vi "IsSearchGoalNode.vi"(8 "error in (no error)":errorcluster, 10 "PossibleGoalNode in":refnum<data-value>, 11 "Graph in":refnum<class "Graph.lvclass">) -> (0 "error out":errorcluster, 1 "IsGoal":bool, 2 "PossibleGoalNode out":refnum<data-value>, 3 "Graph out":refnum<class "Graph.lvclass">)   [LabVIEW 2010, in "Graph.lvclass"]
doc: "Abstract method. Override this VI to implement a search of a tree. This VI is responsible for determining when we have found the node we are searching for."
uses:
  Graph.lvclass
  GraphNode/GraphNode.lvclass
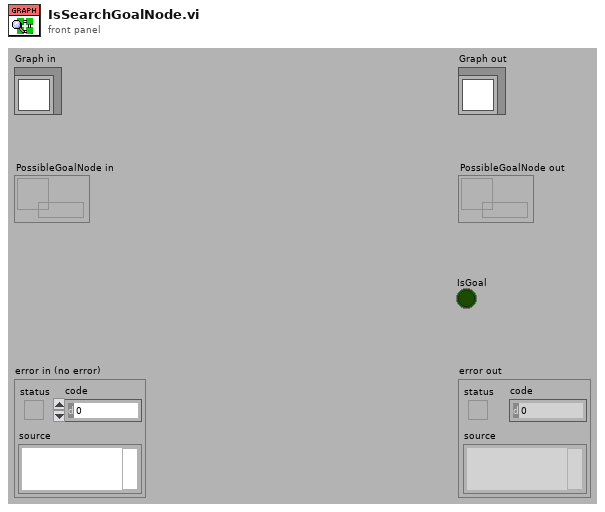
[diagram p1: front panel]
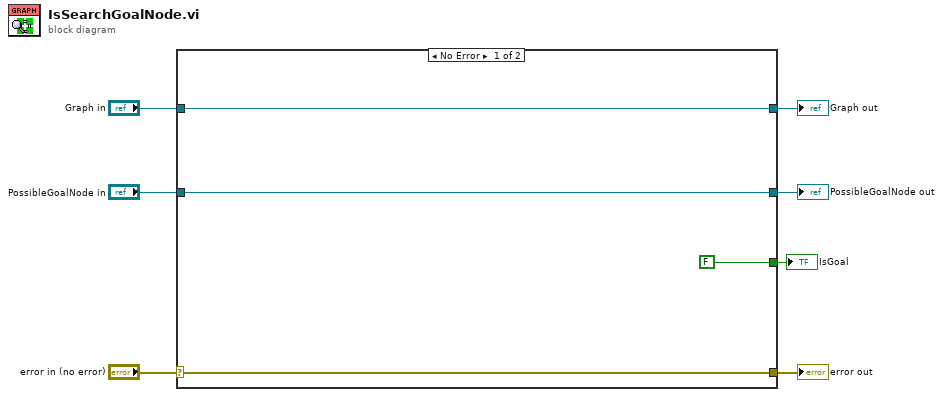
[diagram p0: block diagram]
diagram:
  n1 = case shown="No Error" "error in (no error)" {
    selector: "error in (no error)" -> [w10 w14]
    tunnel: [w10 w14] -> w6
    tunnel: [w11 w13] -> w4
    tunnel: "Graph in" -> [w11 w13]
    tunnel: "PossibleGoalNode in" -> [w9 w12]
    tunnel: [w9 w12] -> w2
    tunnel: [FALSE _] -> w1
    frame No Error {
    }
    frame Error {
    }
  }
  "error out" <- w6
  "Graph out" <- w4
  "PossibleGoalNode out" <- w2
  "IsGoal" <- w1
